vi "Temperature.vi"(2 "°C a °F":bool, 3 "Temperatura":dbl(slide) scale=0.0..1.0) -> (0 "Numeric":dbl, 1 "Termometro":dbl(slide) scale=0.0..250.0)   [LabVIEW 2015]
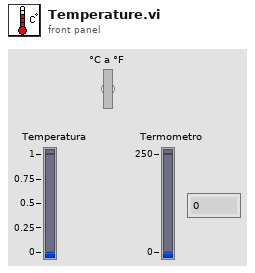
[diagram p1: front panel]
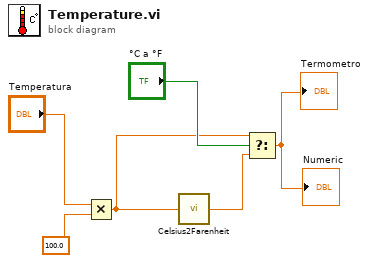
[diagram p0: block diagram]
diagram:
  n1 = Multiply(x="Temperatura", y=100.0) -> (x*y=w2:dbl)
  n2 = call "Celsius2Farenheit.vi"("°C"=w2) -> ("°F"=w1:dbl)
  n3 = Select(t=w2, s="°C a °F", f=w1) -> (s? t:f=→"Termometro" →"Numeric":dbl)
